vi "Get Caraya Library Information.vi"() -> (1 "Library Info":T1, 3 "reserved":refnum<class>)   [LabVIEW 2013, in "Caraya.lvlib"]
uses:
  Caraya.lvlib
  subVIs/Caraya Library Info.ctl
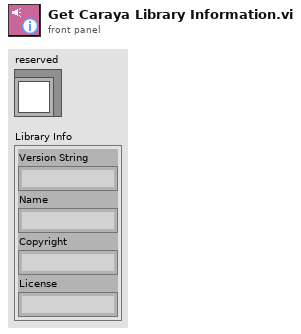
[diagram p1: front panel]
types:
  T1 = typedef "Caraya.lvlib/Caraya Library Info.ctl" = cluster{"Version String":string, "Name":string, "Copyright":string, "License":string}
  T2 = cluster{"Version String":string, "Name":string, "Copyright":string, "License":string}
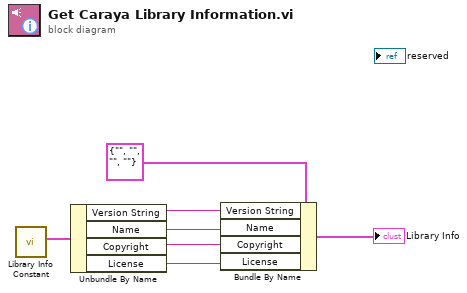
[diagram p0: block diagram]
diagram:
  n1 = call "Library Info Constant.vi"() -> ("Library Info Constant"=w7:T2)  [unwired: 11 in]
  n2 = Unbundle By Name(w7) -> ("Version String"=w5:string, "Name"=w4:string, "Copyright"=w3:string, "License"=w2:string)
  n3 = Bundle By Name(cluster=T1 {"Version String"="", "Name"="", "Copyright"="", "License"=""} ("Caraya Library Info"), "Version String"=w5, "Name"=w4, "Copyright"=w3, "License"=w2) -> (→"Library Info":T1)
